vi "Write Servo Switch.vi"(8 "error in (no error)":errorcluster, 10 "Servo Switch":refnum<class "Servo Switch.lvclass">, 11 "tCRD in":refnum<class "Open Path CRD.lvclass">) -> (0 "error out":errorcluster, 3 "tCRD out":refnum<class "Open Path CRD.lvclass">)   [LabVIEW 2015, in "Open Path CRD.lvclass"]
uses:
  Open Path CRD.lvclass
  Switch/Servo Switch.lvclass
  Open Path CRD.lvclass/Open Path CRD.ctl
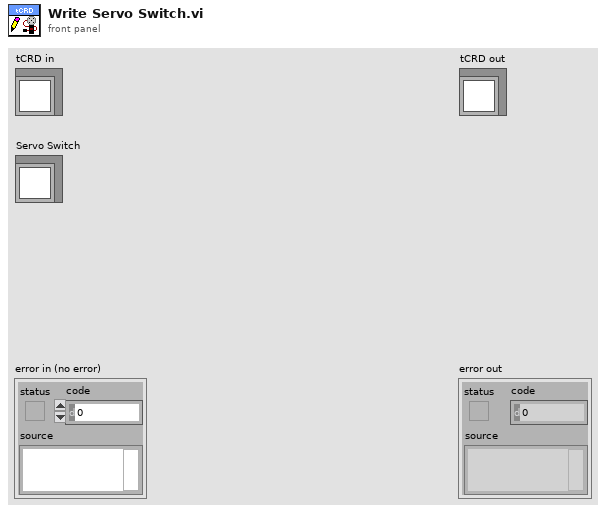
[diagram p1: front panel]
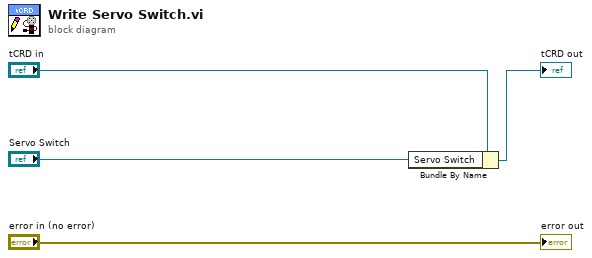
[diagram p0: block diagram]
diagram:
  n1 = Bundle By Name(cluster="tCRD in", "Servo Switch"="Servo Switch") -> (→"tCRD out":refnum<class "Open Path CRD.lvclass">)
  "error out" <- "error in (no error)"
